vi "LECTURA.vi"(0 "File Path":path) -> (1 "lowercase file extension":string, 2 "new picture":picture, 3 "24-bit pixmap":u32[][](array[numeric]))   [LabVIEW 2020]
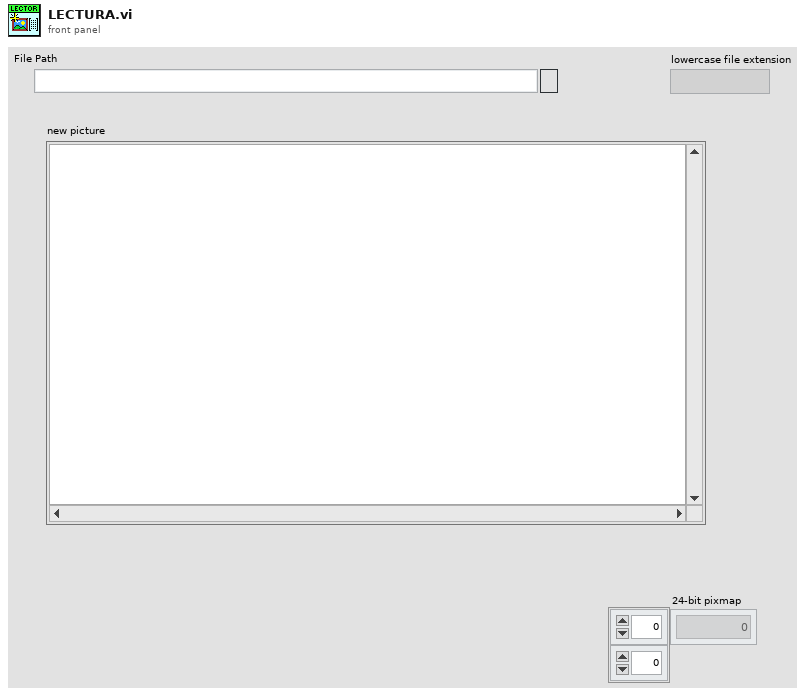
[diagram p1: front panel]
types:
  T1 = typedef "imagedata.ctl" = cluster{"image type":i32, "image depth":i32, "image":u8[], "mask":u8[], "colors":u32[], "Rectangle":cluster{"left":i16, "top":i16, "right":i16, "bottom":i16}}
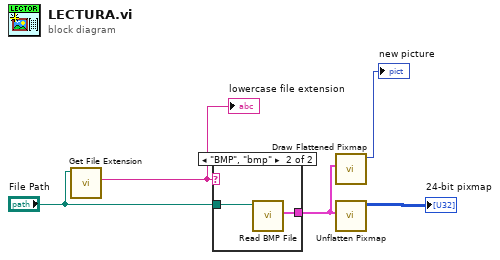
[diagram p0: block diagram]
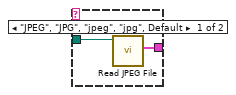
[diagram p2: hidden frame]
diagram:
  n1 = call <vilib>:"Get File Extension.vi"("file"="File Path") -> ("lowercase file extension"=w5:string)  [unwired: 6 in, 4 out]
  "lowercase file extension" <- w5
  n2 = case shown="\"BMP\", \"bmp\"" w5 {
    tunnel: "File Path" -> [w7 w9]
    tunnel: [w6 w8] -> w2
    frame "JPEG", "JPG", "jpeg", "jpg", Default {
      n3 = call <vilib>:"Read JPEG File.vi"("path to JPEG file"=w7) -> ("image data"=w6:T1)  [unwired: 8 in, 2 out]
    }
    frame "BMP", "bmp" {
      n4 = call <vilib>:"Read BMP File.vi"("path to BMP file"=w9) -> ("image data"=w8:T1)  [unwired: 8 in, 2 out]
    }
  }
  n5 = call <vilib>:"Draw Flattened Pixmap.vi"("image data"=w2) -> ("new picture"=→"new picture":picture)  [unwired: 8 in]
  n6 = call <vilib>:"Unflatten Pixmap.vi"("image data"=w2) -> ("24-bit pixmap"=→"24-bit pixmap":u32[][])  [unwired: 4 in, 6 out]
